vi "mWADC_Read.vi"(8 "error in (no error)":errorcluster, 11 "MW_ADC":refnum<visa-resource-name>) -> (0 "error out":errorcluster, 2 "ADC Count":i32, 3 "VISA resource name out":refnum<visa-resource-name>)   [LabVIEW 2019]
panel:
  out "number":i32
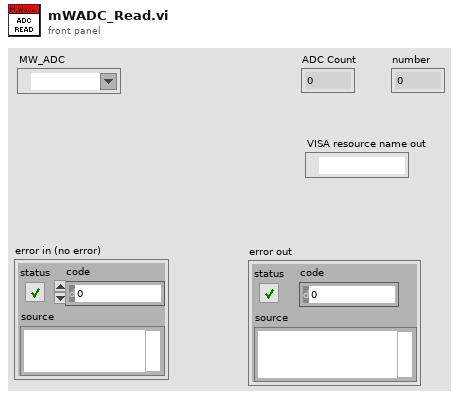
[diagram p1: front panel]
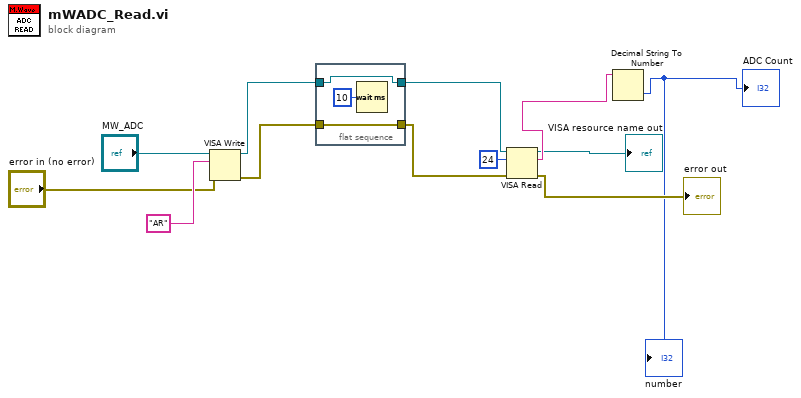
[diagram p0: block diagram]
diagram:
  n1 = VISA Write(VISA resource name="MW_ADC", write buffer="AR", error in (no error)="error in (no error)") -> (VISA resource name out=w11:refnum<visa-resource-name>, error out=w9:errorcluster)  [unwired: 1 out]
  n2 = flat-sequence {
    tunnel: w11 -> [w14]
    tunnel: [w14] -> w10
    tunnel: w9 -> [w13]
    tunnel: [w13] -> w8
    frame #0 {
      n3 = Wait (ms)(milliseconds to wait=u32 10) -> ()  [unwired: 1 out]
    }
  }
  n4 = VISA Read(VISA resource name=w10, byte count=u32 24, error in (no error)=w8) -> (VISA resource name out=→"VISA resource name out":refnum<visa-resource-name>, read buffer=w6:string, error out=→"error out":errorcluster)  [unwired: 1 out]
  n5 = Decimal String To Number(string=w6) -> (number=→"ADC Count" →"number":i32)  [unwired: 2 in, 1 out]
